vi "Radius Search 2D Int.vi"() -> ()   [LabVIEW 2020]
uses:
  <vilib>/numeric/Random Number (Range) I64.vi
  <vilib>/numeric/sub_Random U32.vi
  Classes/KD Tree Int/KD Tree Int.lvclass
  E:/Labview/LV 2020/Libs/flann/flann/Classes/KD Tree/KD Tree.lvclass
  Classes/KD Tree Int/Create KD Tree Int.vi
  Classes/KD Tree Int/Radius Search Int.vi
  Classes/KD Tree/KD Tree.lvclass
panel:
  out "N Found":i32[](array[numeric])
  out "XY Graph":cluster{cluster{i32, i32}[]}[](graph)
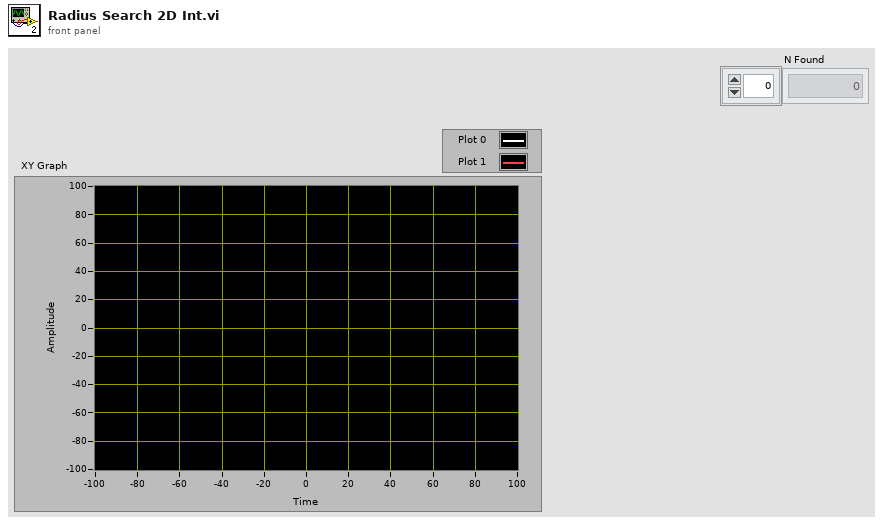
[diagram p1: front panel]
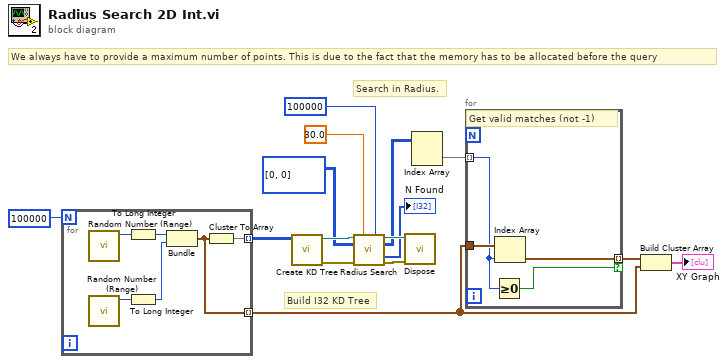
[diagram p0: block diagram]
diagram:
  # "We always have to provide a maximum number of points. This is due to the fact that the memory has to be allocated before the query"
  # "Search in Radius."
  # "Build I32 KD Tree"
  n1 = for {
    N: 100000 -> [_]
    tunnel: [w19] -> w5 mode=indexing
    tunnel: [w18] -> w14 mode=indexing
    n2 = call-poly <vilib>:"Random Number (Range).vi"() -> ("number"=w21:i64)  [unwired: 11 in]
    n3 = call-poly <vilib>:"Random Number (Range).vi"() -> ("number"=w20:i64)  [unwired: 11 in]
    n4 = To Long Integer(number=w21) -> (32bit integer=w17:i32)
    n5 = To Long Integer(number=w20) -> (32bit integer=w16:i32)
    n6 = Bundle(w17, w16) -> (w19:cluster{i32, i32})  [unwired: 1 in]
    n7 = Cluster To Array(cluster=w19) -> (array=w18:i32[])
  }
  n8 = call-poly "Create KD Tree.vi"("Points (Row-Vectors)"=w14) -> ("error out"=w10:errorcluster, "KD Tree Int out"=w13:refnum<class "KD Tree Int.lvclass">)  [unwired: 9 in]
  n9 = call-poly "Radius Search.vi"("KD Tree Int in"=w13, "Radius"=sgl 30.0, "Max Neighbors"=100000, "Points"=i32[][] [[0, 0]], "error in (no error)"=w10) -> ("KD Tree Int out"=w11:refnum<class "KD Tree Int.lvclass">, "Indices"=w8:i32[][], "N Found"=→"N Found":i32[], "error out"=w9:errorcluster)  [unwired: 6 in, 1 out]
  n10 = call "Dispose.vi"("error in (no error)"=w9, "KD Tree in"=w11) -> ()  [unwired: 9 in, 1 out]
  n11 = Index Array(array=w8) -> (element=w6:i32[])  [unwired: 2 in]
  n12 = for {
    tunnel: w5 -> [w25]
    tunnel: w6 -> [w23] mode=indexing
    tunnel: [w24] -> w4 mode=indexing if=w22
    # "Get valid matches (not -1)"
    n13 = Greater Or Equal To 0?(x=w23) -> (x >= 0?=w22:bool)
    n14 = Index Array(array=w25, index=w23) -> (element=w24:cluster{i32, i32})
  }
  n15 = Build Cluster Array(w4, w5) -> (→"XY Graph":cluster{cluster{i32, i32}[]}[])
